vi "interpolate.vi"(0 "Ve_in":dbl[](array[numeric]), 1 "time_in":dbl[](array[numeric])) -> (2 "finalSize":i32, 3 "Ve_out":dbl[](array[numeric]), 4 "time_out":dbl[](array[numeric]))   [LabVIEW 2015]
uses:
  <vilib>/gmath/NI_Gmath.lvlib
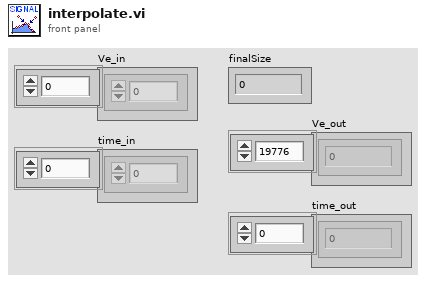
[diagram p1: front panel]
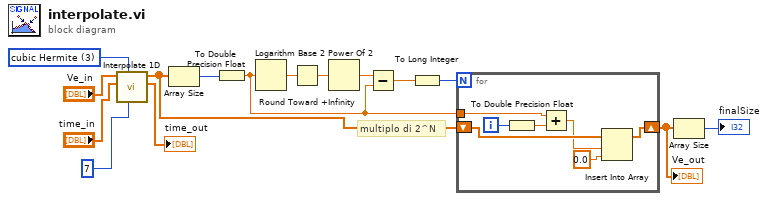
[diagram p0: block diagram]
diagram:
  w8 = 3 items=["nearest", "linear", "spline", "cubic Hermite", "Lagrange"] ("method")
  # "multiplo di 2^N"
  n1 = call <vilib>:"Interpolate 1D.vi"("ntimes"=7, "method"=w8, "X"="time_in", "Y"="Ve_in") -> ("xi used"=→"time_out":dbl[], "yi"=w10:dbl[])  [unwired: 5 in, 1 out]
  n2 = Array Size(array=w10) -> (size(s)=w12:i32)
  n3 = To Double Precision Float(number=w12) -> (double precision float=w7:dbl)
  n4 = Logarithm Base 2(1:w7) -> (0:w2:dbl)
  n5 = Round Toward +Infinity(x=w2) -> (ceil(x): smallest int >= x=w3:dbl)
  n6 = Power Of 2(x=w3) -> (2^x=w4:dbl)
  n7 = Subtract(x=w4, y=w7) -> (x-y=w5:dbl)
  n8 = To Long Integer(number=w5) -> (32bit integer=w6:i32)
  n9 = for {
    N: w6 -> [_]
    shift-right: [w20] -> w13
    shift-left: w10 -> [w22]
    tunnel: w7 -> [w19]
    i -> [w18]
    n10 = To Double Precision Float(number=w18) -> (double precision float=w17:dbl)
    n11 = Add(x=w19, y=w17) -> (x+y=w16:dbl)
    n12 = Insert Into Array(array=w22, index=w16, new element=0.0 ("new element/subarray")) -> (w20:dbl[])
  }
  "Ve_out" <- w13
  n13 = Array Size(array=w13) -> (size(s)=→"finalSize":i32)
